vi "openImage.vi"(8 "error in (no error)":errorcluster, 11 "ImageStreamViewer in":refnum<class "ImageStreamViewer.lvclass">) -> (0 "error out":errorcluster, 3 "ImageStreamViewer out":refnum<class "ImageStreamViewer.lvclass">)   [LabVIEW 2011, in "Views.lvlib" / "Camera.lvlib" / "ImageStreamViewer.lvclass"]
uses:
  ImageStreamViewer.lvclass
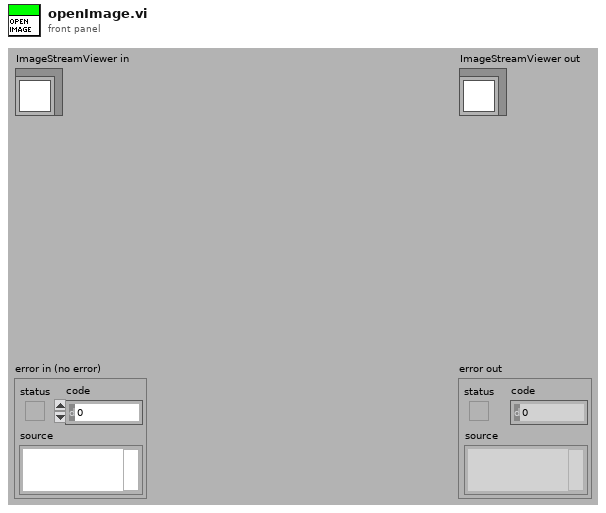
[diagram p1: front panel]
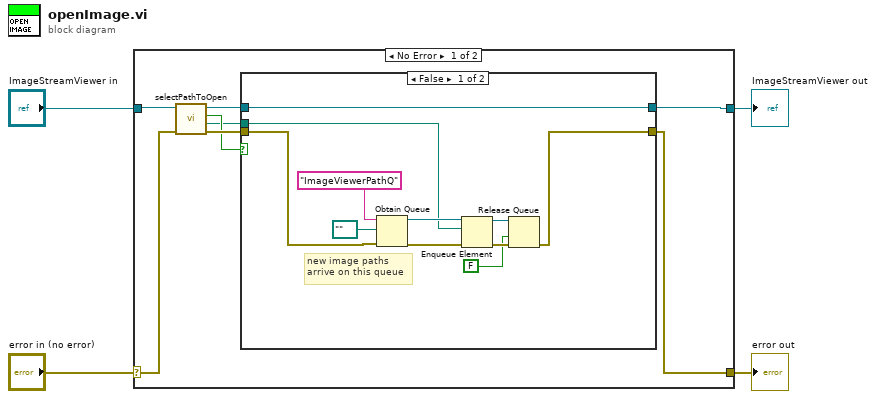
[diagram p0: block diagram]
diagram:
  n1 = case shown="No Error" "error in (no error)" {
    selector: "error in (no error)" -> [w11 w27]
    tunnel: [w6 w27] -> w3
    tunnel: [w7 w26] -> w1
    tunnel: "ImageStreamViewer in" -> [w12 w26]
    frame No Error {
      n2 = call "selectPathToOpen.vi"("error in (no error)"=w11, "ImageStreamViewer in"=w12) -> ("error out"=w9:errorcluster, "selected path"=w5:path, "notSelected?"=w8:bool, "ImageStreamViewer out"=w10:refnum<class "ImageStreamViewer.lvclass">)  [unwired: 6 in]
      n3 = case shown="False" w8 {
        tunnel: w10 -> [w17 w25]
        tunnel: w9 -> [w16 w24]
        tunnel: [w17 w25] -> w7
        tunnel: [w15 w24] -> w6
        tunnel: w5 -> [w19 _]
        frame False {
          # "new image paths\narrive on this queue"
          n4 = Obtain Queue(name (unnamed)="ImageViewerPathQ", element data type=path "", error in (no error)=w16) -> (queue out=w21:refnum<queue>, error out=w20:errorcluster)  [unwired: 2 in, 1 out]
          n5 = Enqueue Element(queue=w21, element=w19, error in (no error)=w20) -> (queue out=w14:refnum<queue>, error out=w18:errorcluster)  [unwired: 1 in, 1 out]
          n6 = Release Queue(queue=w14, force destroy? (F)=FALSE, error in (no error)=w18) -> (error out=w15:errorcluster)  [unwired: 2 out]
        }
        frame True {
        }
      }
    }
    frame Error {
    }
  }
  "error out" <- w3
  "ImageStreamViewer out" <- w1
